vi "Autonomous Independent.vi"() -> ()   [LabVIEW 2012]
doc: "This VI is called when autonomous begins, and will automatically be terminated when autonomous ends. You can carry out timed or sensor driven robot movement independently without needing to return to the caller."
uses:
  <vilib>/Rock Robotics/WPI/RobotDrive/WPI_RobotDriveGetSetRefNum.vi
panel:
  in  "Number Samples to Average 2":u8=1 min=1 max=128
  in  "Minimum Rate 2":dbl=20.0
  in  "Array 2":dbl[][](array[numeric])=[[5.0, 0.0, 20.0, 0.0], [5.0, 90.0, 0.0, 0.0], [5.0, 0.0, 20.0, 0.0], [5.0, 90.0, 0.0, 0.0], [5.0, 0.0, 20.0, 0.0], [5.0, 90.0, 0.0, 0.0], [5.0, 0.0, 20.0, 0.0]]
  out "?":dbl
  out "Distance (in) 4":dbl
  out "?":dbl
  out "Distance (in) 3":dbl
  # "Rotate"
  # "Distance"
  # "Shoot"
  # "Time"
  # "Shoot"
  # "Time"
  # "Rotate"
  # "Distance"
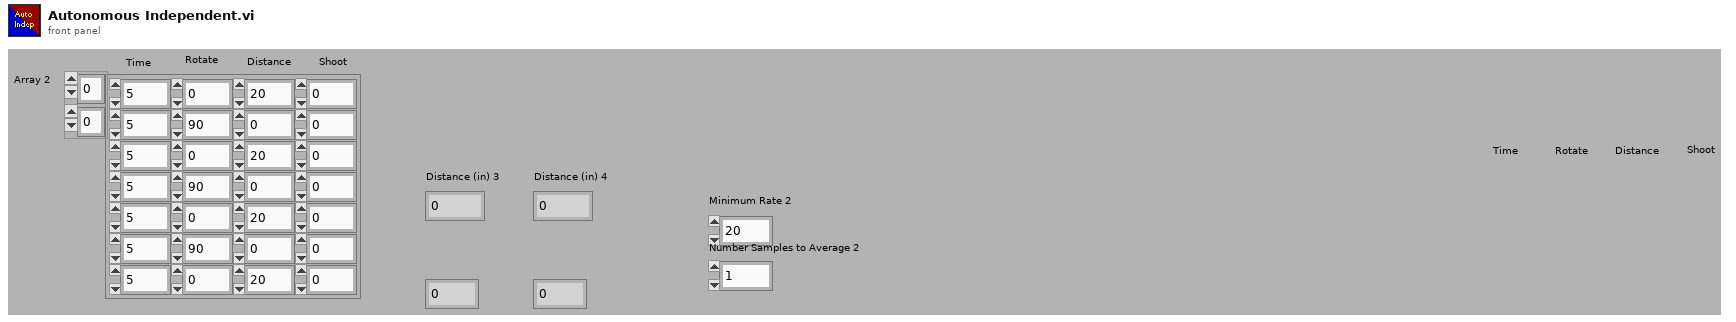
[diagram p1: front panel]
types:
  T1 = typedef "WPI_EncoderDevRef.ctl" = cluster{"DevStatus":errorcluster, "EncoderIndex":T2, "CounterIndex":T3, "DistancePerCount":dbl, "Decoding Type":T4}
  T2 = typedef "FPGA_EncoderIdx.ctl" = enum8{"Enc 0", "Enc 1", "Enc 2", "Enc 3", "Invalid"}
  T3 = typedef "FPGA_CounterCtrSystemIndex.ctl" = enum8{"Ctr 0", "Ctr 1", "Ctr 2", "Ctr 3", "Ctr 4", "Ctr 5", "Ctr 6", "Ctr 7", "Invalid"}
  T4 = typedef "WPI_EncoderType.ctl" = enum16{"1x", "2x", "4x"}
  T5 = typedef "WPI_GyroDevRef.ctl" = cluster{"DevStatus":errorcluster, "Analog Module":T6, "Analog Channel":T7, "Offset":dbl, "Gain (VoltsPerDegree/Second)":dbl}
  T6 = typedef "FPGA_TypedefAnalogModule.ctl" = enum16{"Analog Module 1", "Analog Module 2"}
  T7 = typedef "FPGA_AIChannel.ctl" = enum8{"AI 1", "AI 2", "AI 3", "AI 4", "AI 5", "AI 6", "AI 7", "AI 8", "Invalid"}
  T8 = typedef "WPI_RobotDriveDevRef.ctl" = cluster{"DevStatus":errorcluster, "Motors[]":T9[], "Square Inputs":bool, "Max Output":dbl, "Isochronous":bool}
  T9 = typedef "WPI_MotorControlDeviceRef.ctl" = cluster{"DeviceStatus":errorcluster, "Type":enum16{"PWM", "CAN"}, "PWM":cluster{"Digital Module":T10, "PWM Channel":T11, "DeadBand":T12}, "CAN":cluster{"Device Number":u8, "Control Mode":T13, "Semaphore":T14, "Max Vout":dbl}, "Invert":bool, "TransformRef":T15, "InvTransformRef":T15}
  T10 = typedef "FPGA_TypedefDigitalModule.ctl" = enum16{"Digital Module 1", "Digital Module 2"}
  T11 = typedef "FPGA_DIOPWMChannel.ctl" = enum8{"PWM 1", "PWM 2", "PWM 3", "PWM 4", "PWM 5", "PWM 6", "PWM 7", "PWM 8", "PWM 9", "PWM 10", "Invalid"}
  T12 = typedef "WPI_PWMDeadband.ctl" = cluster{"Name":string, "maxPositivePwm":i32, "minPositivePwm":i32, "centerPwm":i32, "maxNegativePwm":i32, "minNegativePwm":i32, "angularRange":u16}
  T13 = typedef "WPI_CANJaguar_ControlMode.ctl" = enum8{"Percent VBus", "Current", "Speed", "Position", "Voltage"}
  T14 = typedef "Semaphore RefNum" = refnum<k1>
  T15 = typedef "WPI_PWMTransform_ConPane.ctl" = refnum<vi>
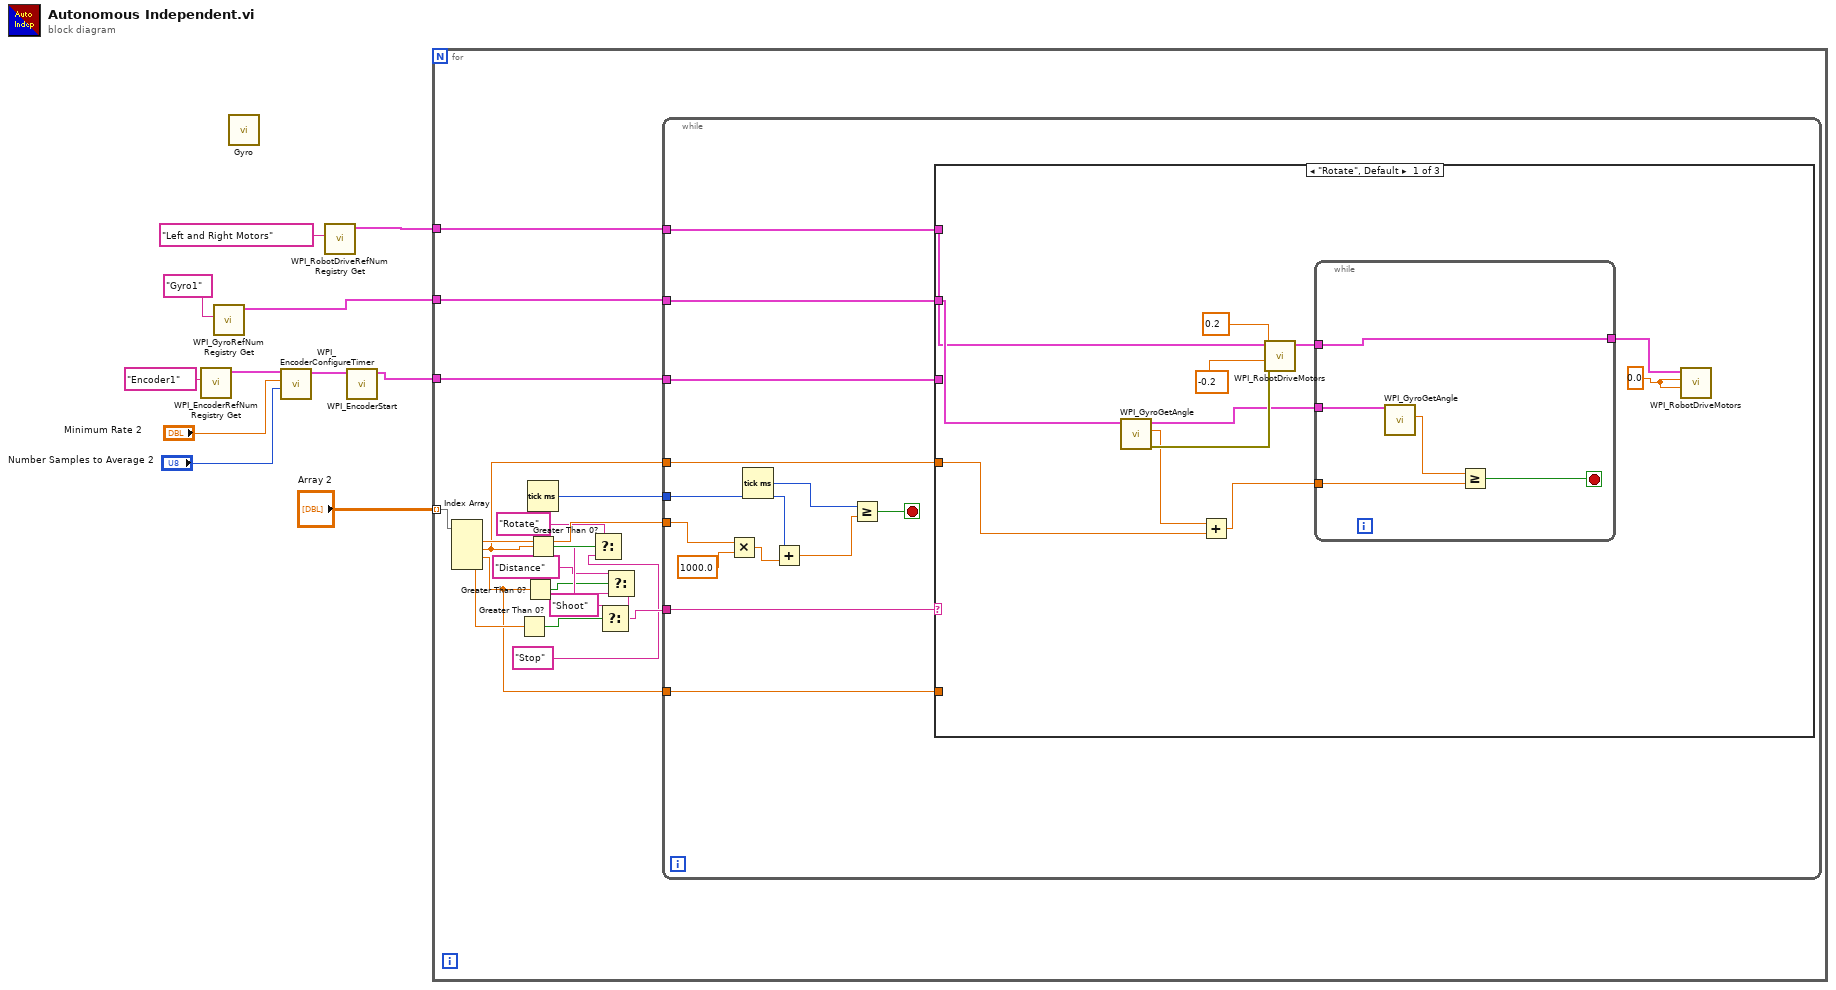
[diagram p0: block diagram]
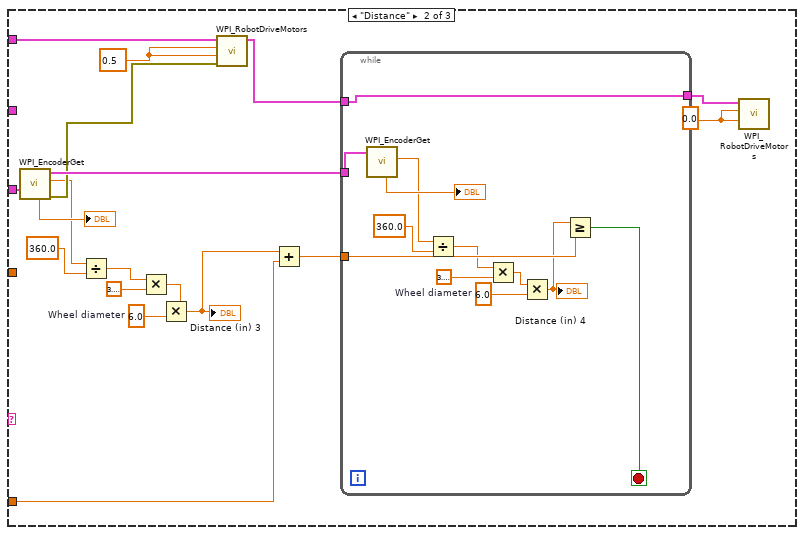
[diagram p2: hidden frame]
diagram:
  n1 = call <vilib>:"WPI_EncoderRefNum Registry Get.vi"("refnum name"="Encoder1") -> ("EncoderDevRef"=w5:T1)  [unwired: 9 in, 1 out]
  n2 = call <vilib>:"WPI_GyroRefNum Registry Get.vi"("refnum name"="Gyro1") -> ("GyroDevRef"=w8:T5)  [unwired: 9 in, 1 out]
  n3 = call "Gyro.vi"() -> ()  [unwired: 1 in]
  n4 = call <vilib>:"WPI_EncoderConfigureTimer.vi"("Number Samples to Average"="Number Samples to Average 2", "Minimum Rate"="Minimum Rate 2", "EncoderDevRef"=w5) -> ("EncoderDevRef"=w2:T1)  [unwired: 1 in, 7 out]
  n5 = call <vilib>:"WPI_RobotDriveRefNum Registry Get.vi"("refnum name"="Left and Right Motors") -> ("RobotDriveDevRef"=w10:T8)  [unwired: 9 in, 1 out]
  n6 = call <vilib>:"WPI_EncoderStart.vi"("EncoderDevRef"=w2) -> ("EncoderDevRef"=w1:T1)  [unwired: 1 in, 9 out]
  n7 = for {
    tunnel: w10 -> [w30]
    tunnel: w8 -> [w29]
    tunnel: w1 -> [w28]
    tunnel: "Array 2" -> [w27] mode=indexing
    n8 = Index Array(array=w27) -> (element #1=w26:dbl, element #2=w13:dbl, element #3=w12:dbl, element #4=w18:dbl)  [unwired: 4 in]
    n9 = Greater Than 0?(x=w18) -> (x > 0?=w19:bool)
    n10 = Greater Than 0?(x=w12) -> (x > 0?=w20:bool)
    n11 = Tick Count (ms)() -> (millisecond timer value=w25:u32)
    n12 = Greater Than 0?(x=w13) -> (x > 0?=w24:bool)
    n13 = Select(t="Rotate", s=w24, f="Stop") -> (s? t:f=w22:string)
    n14 = Select(t="Distance", s=w20, f=w22) -> (s? t:f=w21:string)
    n15 = Select(t="Shoot", s=w19, f=w21) -> (s? t:f=w15:string)
    n16 = while {
      tunnel: w30 -> [w42]
      tunnel: w29 -> [w43]
      tunnel: w28 -> [w41]
      tunnel: w26 -> [w39]
      tunnel: w25 -> [w38]
      tunnel: w15 -> [w33]
      tunnel: w13 -> [w32]
      tunnel: w12 -> [w31]
      stop <- w34 stop-if-true
      n17 = Multiply(x=w39, y=1000.0) -> (x*y=w37:dbl)
      n18 = Tick Count (ms)() -> (millisecond timer value=w36:u32)
      n19 = Add(x=w38, y=w37) -> (x+y=w35:dbl)
      n20 = Greater Or Equal?(x=w36, y=w35) -> (x >= y?=w34:bool)
      n21 = case shown="\"Rotate\", Default" w33 {
        tunnel: w43 -> [w55 _ _]
        tunnel: w42 -> [w51 w78 _]
        tunnel: w41 -> [_ w64 _]
        tunnel: w32 -> [w44 _ _]
        tunnel: w31 -> [_ w61 _]
        frame "Rotate", Default {
          w46 = 0.0 ("LeftSpeed")
          n22 = call <vilib>:"WPI_GyroGetAngle.vi"("GyroDevRef"=w55) -> ("error out"=w54:errorcluster, "Angle"=w50:dbl, "GyroDevRef"=w45:T5)  [unwired: 7 in, 1 out]
          n23 = Add(x=w50, y=w44) -> (x+y=w49:dbl)
          n24 = call <vilib>:"WPI_RobotDriveMotors.vi"("error in (no error)"=w54, "RightSpeed"=-0.2, "LeftSpeed"=0.2, "RobotDriveDevRef"=w51) -> ("RobotDriveDevRef"=w48:T8)  [unwired: 5 in, 2 out]
          n25 = while {
            tunnel: w49 -> [w59]
            tunnel: w48 -> [w58]
            tunnel: [w58] -> w47
            tunnel: w45 -> [w57]
            stop <- w56 stop-if-true
            n26 = call <vilib>:"WPI_GyroGetAngle.vi"("GyroDevRef"=w57) -> ("Angle"=w60:dbl)  [unwired: 7 in, 3 out]
            n27 = Greater Or Equal?(x=w60, y=w59) -> (x >= y?=w56:bool)
          }
          n28 = call <vilib>:"WPI_RobotDriveMotors.vi"("RightSpeed"=w46, "LeftSpeed"=w46, "RobotDriveDevRef"=w47) -> ()  [unwired: 6 in, 3 out]
        }
        frame "Distance" {
          w72 = 6.0  # Wheel diameter
          w73 = 0.0
          w77 = 0.5
          n29 = call <vilib>:"WPI_EncoderGet.vi"("EncoderDevRef"=w64) -> ("error out"=w65:errorcluster, "Distance"=w63:dbl, "EncoderDevRef"=w66:T1, "Rate"=→"?":dbl)  [unwired: 1 in, 6 out]
          n30 = Divide(x=w63, y=360.0) -> (x/y=w67:dbl)
          n31 = Multiply(x=w67, y=3.141592653589793) -> (x*y=w68:dbl)
          n32 = Multiply(x=w68, y=w72) -> (x*y=w62:dbl)
          "Distance (in) 3" <- w62
          n33 = call <vilib>:"WPI_RobotDriveMotors.vi"("error in (no error)"=w65, "RightSpeed"=w77, "LeftSpeed"=w77, "RobotDriveDevRef"=w78) -> ("RobotDriveDevRef"=w76:T8)  [unwired: 5 in, 2 out]
          n34 = Add(x=w62, y=w61) -> (x+y=w74:dbl)
          n35 = while {
            tunnel: w76 -> [w90]
            tunnel: [w90] -> w75
            tunnel: w74 -> [w89]
            tunnel: w66 -> [w82]
            stop <- w84 stop-if-true
            w85 = 6.0  # Wheel diameter
            n36 = call <vilib>:"WPI_EncoderGet.vi"("EncoderDevRef"=w82) -> ("Distance"=w80:dbl, "Rate"=→"?":dbl)  [unwired: 1 in, 8 out]
            n37 = Divide(x=w80, y=360.0) -> (x/y=w88:dbl)
            n38 = Multiply(x=w88, y=3.141592653589793) -> (x*y=w83:dbl)
            n39 = Multiply(x=w83, y=w85) -> (x*y=w79:dbl)
            "Distance (in) 4" <- w79
            n40 = Greater Or Equal?(x=w79, y=w89) -> (x >= y?=w84:bool)
          }
          n41 = call <vilib>:"WPI_RobotDriveMotors.vi"("RightSpeed"=w73, "LeftSpeed"=w73, "RobotDriveDevRef"=w75) -> ()  [unwired: 6 in, 3 out]
        }
        frame "Shoot" {
        }
      }
    }
  }
